vi "NoServicesRegistered_InvalidRegisterRequests_Error.vi"() -> (6 "pass":bool, 8 "result":string, 15 "error out":errorcluster)   [LabVIEW 2020]
uses:
  Runtime/MeasurementLink Discovery Client/RPC Messages/ni_measurementlink_discovery_v1_RegisterServiceRequest.ctl
  Runtime/MeasurementLink Discovery Client/RPC Messages/ni_measurementlink_discovery_v1_ServiceDescriptor.ctl
  Runtime/MeasurementLink Discovery Client/RPC Messages/ni_measurementlink_discovery_v1_ServiceDescriptor_AnnotationsEntry.ctl
  Runtime/MeasurementLink Discovery Client/RPC Messages/ni_measurementlink_discovery_v1_ServiceLocation.ctl
  <vilib>/ErrorRing/Error Ring.xnode
  Runtime/MeasurementLink Discovery Client/MeasurementLink Discovery Client.lvlib
  Runtime/MeasurementLink Discovery V1/MeasurementLink Discovery V1.lvlib
panel:
  # "Test assumes discovery service has already been started."
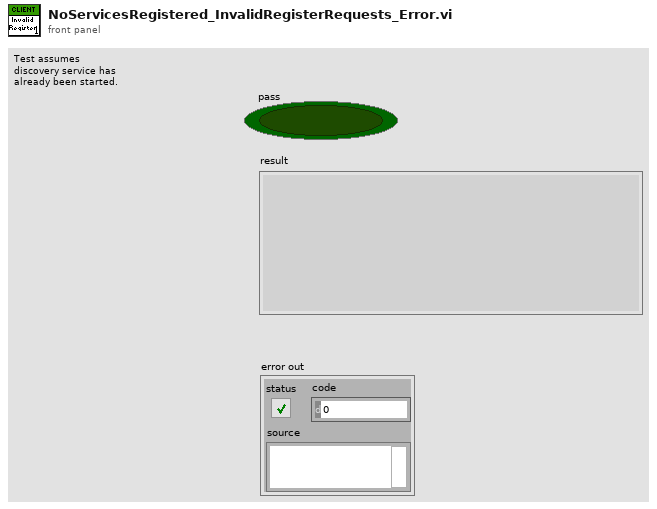
[diagram p1: front panel]
types:
  T1 = typedef "MeasurementLink Discovery Client.lvlib/ni_measurementlink_discovery_v1_RegisterServiceRequest.ctl" = cluster{"service_description":T2, "location":T4}
  T2 = typedef "MeasurementLink Discovery Client.lvlib/ni_measurementlink_discovery_v1_ServiceDescriptor.ctl" = cluster{"display_name":string, "description_url":string, "provided_interfaces":string[], "service_class":string, "annotations":T3[]}
  T3 = typedef "MeasurementLink Discovery Client.lvlib/ni_measurementlink_discovery_v1_ServiceDescriptor_AnnotationsEntry.ctl" = cluster{"key":string, "value":string}
  T4 = typedef "MeasurementLink Discovery Client.lvlib/ni_measurementlink_discovery_v1_ServiceLocation.ctl" = cluster{"location":string, "insecure_port":string, "ssl_authenticated_port":string}
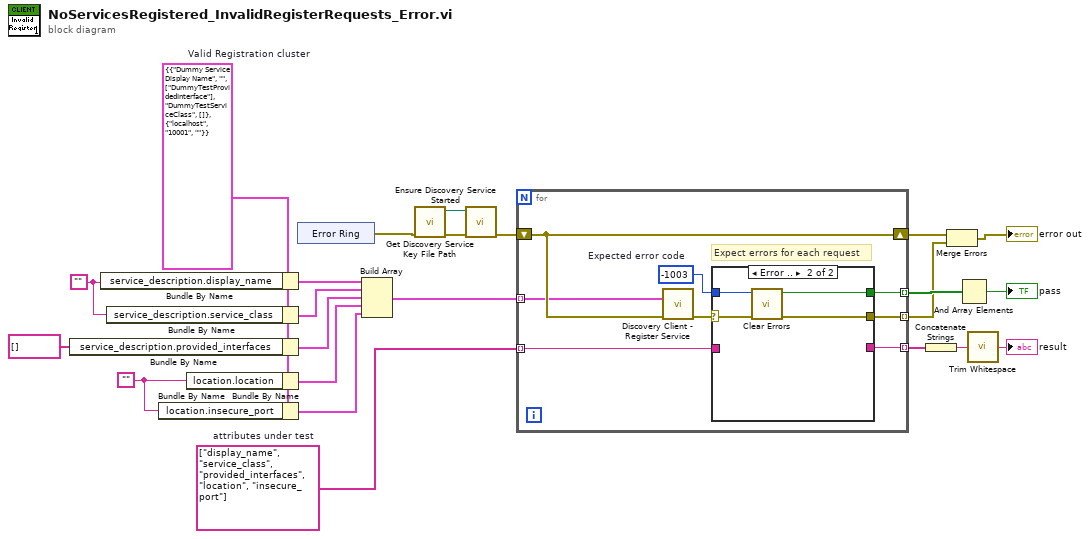
[diagram p0: block diagram]
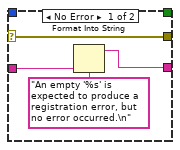
[diagram p2: hidden frame]
diagram:
  w8 = string[] ["display_name", "service_class", "provided_interfaces", "location", "insecure_port"]  # attributes under test
  w14 = ""
  w19 = ""
  w13 = T1 {"service_description"={"display_name"="Dummy Service Display Name", "description_url"="", "provided_interfaces"=["DummyTestProvidedInterface"], "service_class"="DummyTestServiceClass", "annotations"=[]}, "location"={"location"="localhost", "insecure_port"="10001", "ssl_authenticated_port"=""}}  # Valid Registration cluster
  n1 = Bundle By Name(cluster=w13, "service_description.provided_interfaces"=string[] []) -> (w17:T1)
  n2 = Bundle By Name(cluster=w13, "service_description.display_name"=w19) -> (w20:T1)
  n3 = Bundle By Name(cluster=w13, "service_description.service_class"=w19) -> (w18:T1)
  n4 = Bundle By Name(cluster=w13, "location.insecure_port"=w14) -> (w12:T1)
  n5 = Bundle By Name(cluster=w13, "location.location"=w14) -> (w15:T1)
  n6 = xnode "Error Ring"() -> ("error out"=w3:errorcluster)
  n7 = Build Array(w20, w18, w17, w15, w12) -> (w21:T1[])
  n8 = call "Get Discovery Service Key File Path.vi"("error in"=w3) -> ("error out"=w2:errorcluster, "key file path"=w1:path)  [unwired: 9 in]
  n9 = call "Ensure Discovery Service Started.vi"("error in"=w2, "path"=w1) -> ("error out"=w4:errorcluster)  [unwired: 8 in, 1 out]
  n10 = for {
    tunnel: [w29] -> w22 mode=indexing
    tunnel: w21 -> [w30] mode=indexing
    shift-right: [w31] -> w11
    shift-left: w4 -> [w31]
    tunnel: [w28] -> w9 mode=indexing
    tunnel: w8 -> [w25] mode=indexing
    tunnel: [w24] -> w7 mode=indexing
    w27 = -1003  # Expected error code
    # "Expect errors for each request"
    n11 = call "Discovery Client - Register Service.vi"("Request Data"=w30, "error in (no error)"=w31) -> ("error out"=w26:errorcluster)  [unwired: 12 in, 1 out]
    n12 = case shown="Error .." w26 {
      selector: w26 -> [w35 w36]
      tunnel: [_ w39] -> w29
      tunnel: [w35 w38] -> w28
      tunnel: w27 -> [_ w37]
      tunnel: w25 -> [w34 _]
      tunnel: [w32 _] -> w24
      frame No Error {
        n13 = Format Into String(format string="An empty '%s' is expected to produce a registration error, but no error occurred.\n", w34) -> (resulting string=w32:string)  [unwired: 2 in, 1 out]
      }
      frame Error {
        n14 = call <vilib>:"Clear Errors.vi"("error in (no error)"=w36, "specific error code to clear (0: all)"=w37) -> ("error out"=w38:errorcluster, "specific error cleared?"=w39:bool)  [unwired: 4 in]
      }
    }
  }
  n15 = Concatenate Strings(w7) -> (w6:string)
  n16 = Merge Errors(w11, w9) -> (→"error out":errorcluster)
  n17 = And Array Elements(Boolean array=w22) -> (logical AND=→"pass":bool)
  n18 = call <vilib>:"Trim Whitespace.vi"("string"=w6) -> ("trimmed string"=→"result":string)  [unwired: 1 in]
